vi "_getDPExtByName.vi"(10 "DataPlugin Information":T1[](array[typedef]), 11 "DataPlugin name":string) -> (1 "read-only":bool, 2 "file extensions":string[](array[string]))   [LabVIEW 2020]
uses:
  <vilib>/Platform/storage/utility/usiPluginInformation.ctl
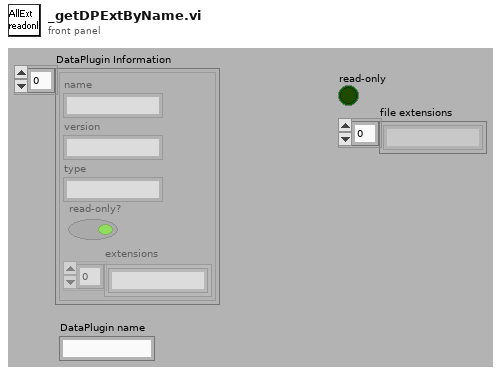
[diagram p1: front panel]
types:
  T1 = typedef "usiPluginInformation.ctl" = cluster{"name":string, "version":string, "type":string, "read-only?":bool, "extensions":string[]}
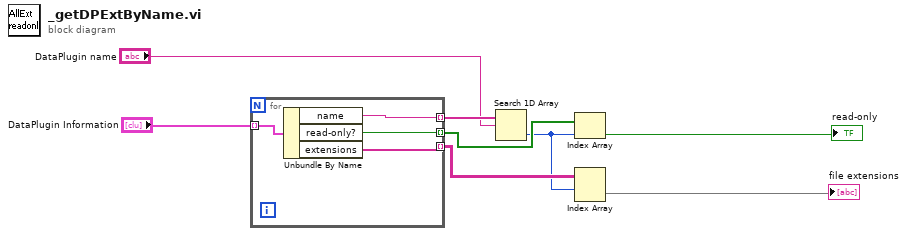
[diagram p0: block diagram]
diagram:
  n1 = for {
    tunnel: "DataPlugin Information" -> [w12] mode=indexing
    tunnel: [w11] -> w7 mode=indexing
    tunnel: [w10] -> w5 mode=indexing
    tunnel: [w9] -> w3 mode=indexing
    n2 = Unbundle By Name(w12) -> ("name"=w11:string, "read-only?"=w10:bool, "extensions"=w9:string[])
  }
  n3 = Search 1D Array(1D array=w7, element="DataPlugin name") -> (index of element=w1:i32)  [unwired: 1 in]
  n4 = Index Array(array=w5, index=w1) -> (element=→"read-only":bool)
  n5 = Index Array(array=w3, index (row)=w1) -> (element=→"file extensions":string[])  [unwired: 1 in]
